vi "FTW-STR-UTF8.vi"(0 "Input":string, 1 "Direction":T1) -> (2 "Output":string)   [LabVIEW 2014]
uses:
  string/FTW-STR-EncodingDirection.ctl
panel:
  # "Inputs"
  # "Outputs"
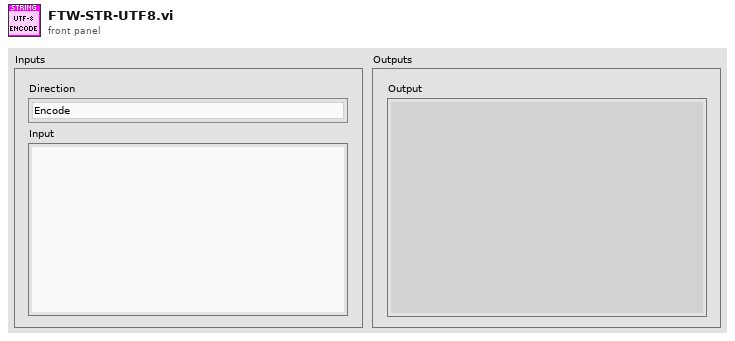
[diagram p1: front panel]
types:
  T1 = typedef "FTW-STR-EncodingDirection.ctl" = enum16{"Encode", "Decode"}
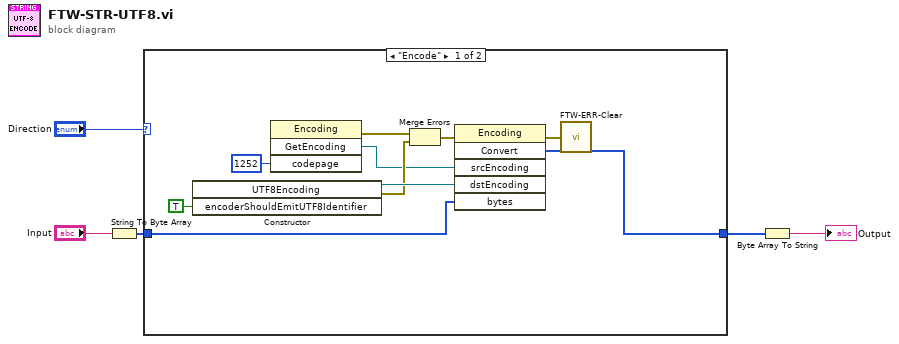
[diagram p0: block diagram]
diagram:
  n1 = String To Byte Array(string="Input") -> (unsigned byte array=w3:u8[])
  n2 = case shown="\"Encode\"" "Direction" {
    tunnel: [w14 w16] -> w4
    tunnel: w3 -> [w13 w16]
    frame "Encode" {
      n3 = constructor class="UTF8Encoding"("encoderShouldEmitUTF8Identifier"=TRUE) -> (reference out=w15:refnum<k24>, error out=w10:errorcluster)  [unwired: 3 in, 2 out]
      n4 = invoke class="Encoding" method="GetEncoding"("codepage"=1252) -> (error out=w6:errorcluster, "GetEncoding"=w7:refnum<k24>)  [unwired: 3 in, 2 out]
      n5 = Merge Errors(w6, w10) -> (w12:errorcluster)
      n6 = invoke class="Encoding" method="Convert"(error in=w12, "srcEncoding"=w7, "dstEncoding"=w15, "bytes"=w13) -> (error out=w11:errorcluster, "Convert"=w14:u8[])  [unwired: 2 in, 4 out]
      n7 = call "FTW-ERR-Clear.vi"("error to snuff"=w11) -> ()  [unwired: 1 out]
    }
    frame "Decode" {
      # "Not yet implemented."
    }
  }
  n8 = Byte Array To String(unsigned byte array=w4) -> (string=→"Output":string)
